vi "F5xxx_wait_for_settle.vi"(8 "error in (no error)":errorcluster, 10 "timeout [ms]":u32=7000, 11 "VISA Refnum in":refnum<visa-resource-name>) -> (0 "error out":errorcluster, 2 "settled":bool, 3 "VISA Refnum out":refnum<visa-resource-name>)   [LabVIEW 2013, in "Fluke 5XXX Series Multicalibrators.lvlib"]
uses:
  Fluke 5XXX Series Multicalibrators.lvlib
panel:
  out "x-y":u32
  out "number":i32 format="%016b"
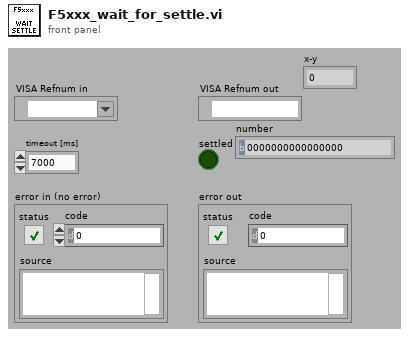
[diagram p1: front panel]
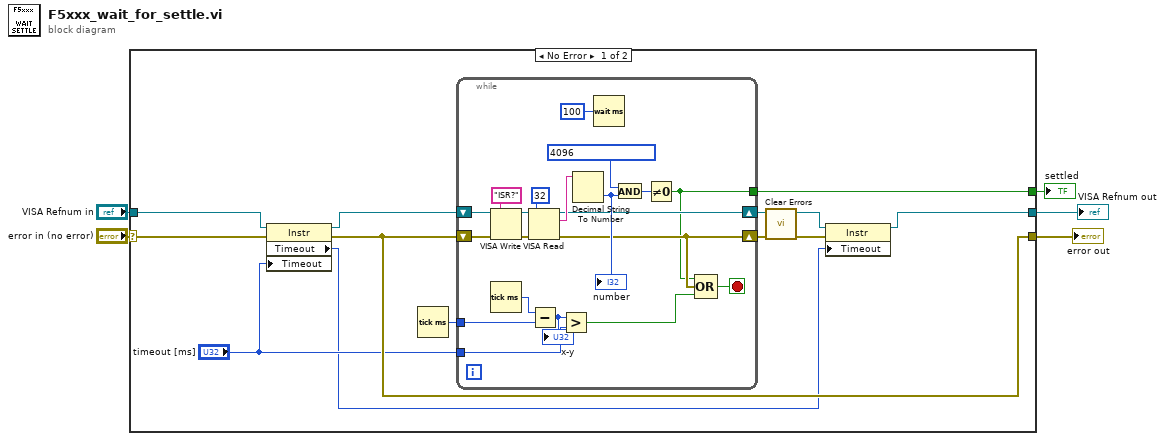
[diagram p0: block diagram]
diagram:
  n1 = case shown="No Error" "error in (no error)" {
    selector: "error in (no error)" -> [w15 w38]
    tunnel: "VISA Refnum in" -> [w12 w39]
    tunnel: [w13 w38] -> w3
    tunnel: [w7 w39] -> w4
    tunnel: [w14 _] -> w1
    frame No Error {
      n2 = property class="Instr"(reference=w12, error in=w15, "Timeout"="timeout [ms]") -> (reference out=w11:refnum<visa-resource-name>, error out=w13:errorcluster, "Timeout"=w6:u32)
      n3 = Tick Count (ms)() -> (millisecond timer value=w17:u32)
      n4 = while {
        shift-right: [w24] -> w16
        shift-left: w13 -> [w37]
        shift-right: [w28] -> w8
        shift-left: w11 -> [w35]
        tunnel: w17 -> [w22]
        tunnel: "timeout [ms]" -> [w20]
        tunnel: [w18] -> w14
        stop <- w25 stop-if-true
        n5 = VISA Write(VISA resource name=w35, write buffer="ISR?", error in (no error)=w37) -> (VISA resource name out=w34:refnum<visa-resource-name>, error out=w36:errorcluster)  [unwired: 1 out]
        n6 = Tick Count (ms)() -> (millisecond timer value=w23:u32)
        n7 = VISA Read(VISA resource name=w34, byte count=u32 32, error in (no error)=w36) -> (VISA resource name out=w28:refnum<visa-resource-name>, read buffer=w31:string, error out=w24:errorcluster)  [unwired: 1 out]
        n8 = Subtract(x=w23, y=w22) -> (x-y=w21:u32)
        "x-y" <- w21
        n9 = Greater?(x=w21, y=w20) -> (0:w19:bool)
        n10 = Decimal String To Number(string=w31) -> (number=w30:i32)  [unwired: 2 in, 1 out]
        "number" <- w30
        n11 = Wait (ms)(milliseconds to wait=u32 100) -> ()  [unwired: 1 out]
        n12 = And(x=4096, y=w30) -> (x .and. y?=w27:i32)
        n13 = Not Equal To 0?(x=w27) -> (x != 0?=w18:bool)
        n14 = Compound Arithmetic op=OR(w18, w24, w19) -> (w25:bool)
      }
      n15 = call <vilib>:"Clear Errors.vi"("error in (no error)"=w16) -> ("error out"=w9:errorcluster)  [unwired: 6 in]
      n16 = property class="Instr"(reference=w8, error in=w9, "Timeout"=w6) -> (reference out=w7:refnum<visa-resource-name>)  [unwired: 1 out]
    }
    frame Error {
    }
  }
  "VISA Refnum out" <- w4
  "error out" <- w3
  "settled" <- w1
